vi "CRYWindow Wait Bridge.vi"(8 "sName":string) -> ()   [LabVIEW 2013]
uses:
  SubVI/CRYMain Sub Window Global.vi
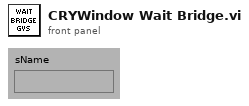
[diagram p1: front panel]
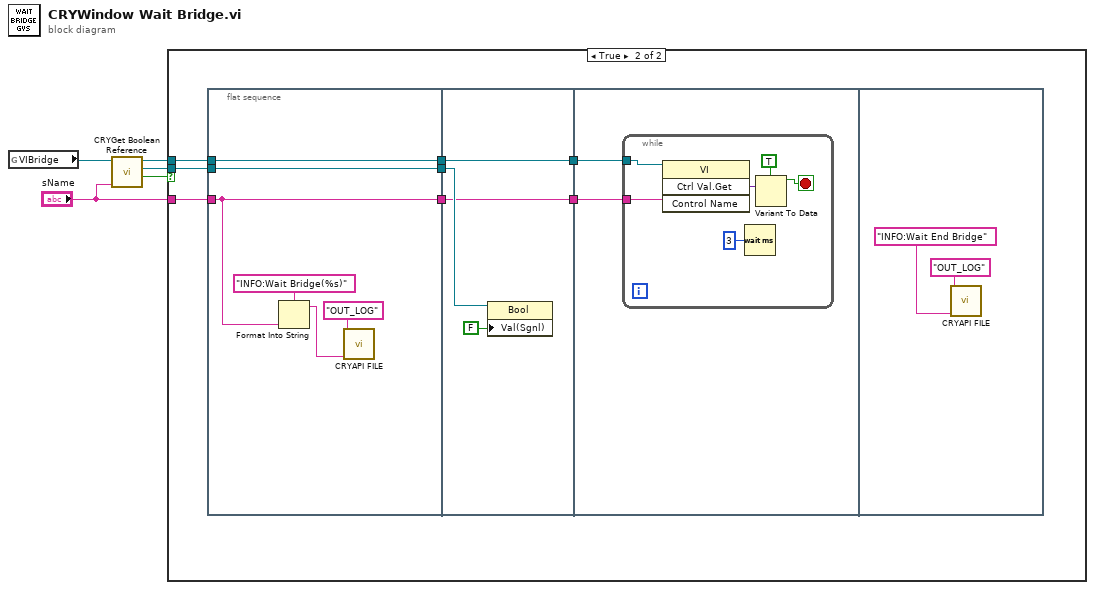
[diagram p0: block diagram]
diagram:
  n1 = global read "CRYMain Sub Window Global.vi" "VIBridge"() -> (w2:refnum<vi>)
  n2 = call "CRYGet Boolean Reference.vi"("Label Name"="sName", "VI Refnum"=w2) -> ("Exist?"=w5:bool, "Boolean Ref"=w4:refnum<vi>, "VI Refnum Out"=w3:refnum<vi>)  [unwired: 7 in]
  n3 = case shown="True" w5 {
    tunnel: w4 -> [_ w13]
    tunnel: w3 -> [_ w12]
    tunnel: "sName" -> [_ w8]
    frame False {
    }
    frame True {
      n4 = flat-sequence {
        tunnel: w12 -> [w18]
        tunnel: w13 -> [w19]
        tunnel: [w19] -> w10
        tunnel: [w18] -> w9
        tunnel: w8 -> [w14]
        tunnel: [w14] -> w6
        tunnel: [w21] -> w11
        tunnel: w10 -> [w23]
        tunnel: w9 -> [w21]
        tunnel: [w20] -> w7
        tunnel: w6 -> [w20]
        tunnel: w11 -> [w25]
        tunnel: w7 -> [w24]
        frame #0 {
          n5 = Format Into String(format string="INFO:Wait Bridge(%s)" ("sAction"), w14) -> (resulting string=w15:string)  [unwired: 2 in, 1 out]
          n6 = call "CRYAPI FILE.vi"("sData"=w15, "sAction"="OUT_LOG") -> ()  [unwired: 8 in, 2 out]
        }
        frame #1 {
          n7 = property class="Bool"(reference=w23, "Val(Sgnl)"=FALSE) -> ()  [unwired: 1 in, 2 out]
        }
        frame #2 {
          n8 = while {
            tunnel: w25 -> [w31]
            tunnel: w24 -> [w27]
            stop <- w28 stop-if-true
            n9 = invoke class="VI" method="Ctrl Val.Get"(reference=w31, "Control Name"=w27) -> ("Get Control Value Variant"=w30:variant)  [unwired: 2 in, 3 out]
            n10 = Wait (ms)(milliseconds to wait=u32 3) -> ()  [unwired: 1 out]
            n11 = Variant To Data(type=TRUE, Variant=w30) -> (data=w28:bool)  [unwired: 1 in, 1 out]
          }
        }
        frame #3 {
          n12 = call "CRYAPI FILE.vi"("sData"="INFO:Wait End Bridge" ("sAction"), "sAction"="OUT_LOG") -> ()  [unwired: 8 in, 2 out]
        }
      }
    }
  }
